vi "Init.vi"(8 "error in (no error)":errorcluster) -> (0 "error out":errorcluster, 3 "Message Queues out":T1)   [LabVIEW 2017]
doc: "This VI creates all Message Queues and User Events, initializes the ErrorHandler and the Stop-Global Variable."
uses:
  SubLibs/Message Queue/CommReferences.ctl
  SubLibs/Message Queue/MessageCluster.ctl
  ServerGlobals.vi
  SubLibs/Message Queue/Message Queue.lvlib
  SubLibs/ErrorLogger/ErrorLogger.lvlib
  Server.lvlib
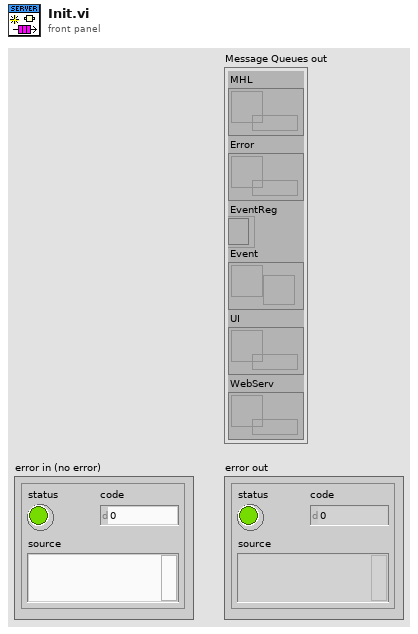
[diagram p1: front panel]
types:
  T1 = typedef "Server.lvlib/Message Queue.lvlib/CommReferences.ctl" = cluster{"MHL":refnum<queue>, "Error":refnum<queue>, "EventReg":refnum<event-registration>, "Event":refnum<user-event>, "UI":refnum<queue>, "WebServ":refnum<queue>}
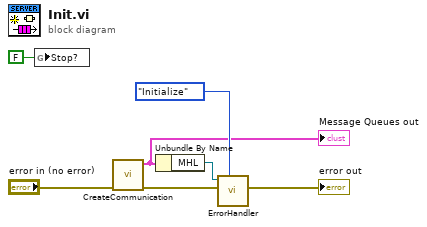
[diagram p0: block diagram]
diagram:
  n1 = global write "ServerGlobals.vi" "Stop?"(FALSE ("Stop?")) -> ()
  n2 = call "CreateCommunication.vi"("error in (no error)"="error in (no error)") -> ("error out"=w6:errorcluster, "Message Queues out"=w2:T1)  [unwired: 9 in]
  "Message Queues out" <- w2
  n3 = Unbundle By Name(w2) -> ("MHL"=w1:refnum<queue>)
  n4 = call "ErrorHandler.vi"("Command(CheckErrors)"=enum16{"Initialize", "CheckErrors"}."Initialize", "Error In"=w6, "MHL"=w1) -> ("Error Out"=→"error out":errorcluster)  [unwired: 8 in]
